vi "Timer.vi"(9 "Timer.Timer enable":bool, 10 "Timer.Tiempo deseado":dbl format="%#_13g", 11 "Class 2.lvclass":refnum<class "Class 2.lvclass">) -> (1 "Timer.Timer DN":bool, 2 "Numeric":dbl, 3 "Class 2.lvclass 2":refnum<class "Class 2.lvclass">)   [LabVIEW 2019, in "Class 2.lvclass"]
uses:
  Class 2.lvclass
  Class 2.lvclass/Class 2.ctl
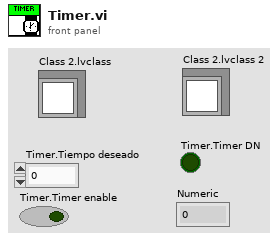
[diagram p1: front panel]
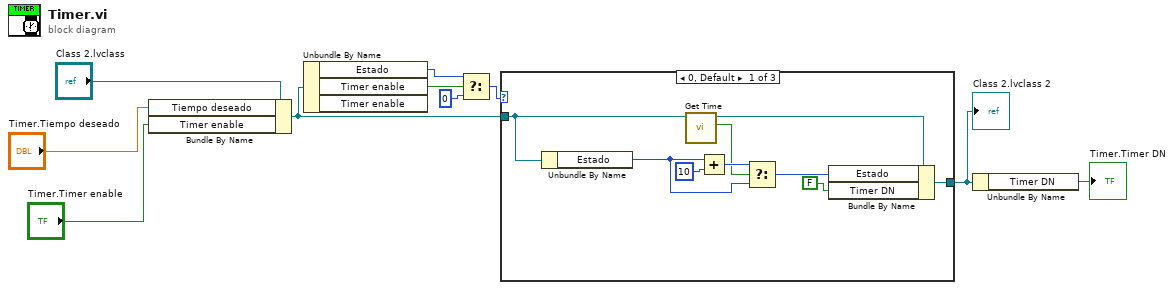
[diagram p0: block diagram]
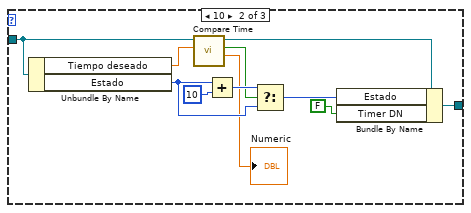
[diagram p2: hidden frame]
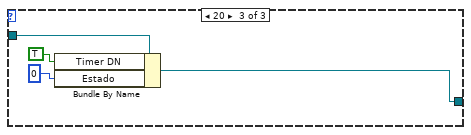
[diagram p3: hidden frame]
diagram:
  n1 = Bundle By Name(cluster="Class 2.lvclass", "Tiempo deseado"="Timer.Tiempo deseado", "Timer enable"="Timer.Timer enable") -> (w8:refnum<class "Class 2.lvclass">)
  n2 = Unbundle By Name(w8) -> ("Estado"=w4:u8, "Timer enable"=w3:bool)  [unwired: 1 out]
  n3 = Select(t=w4, s=w3, f=u8 0) -> (s? t:f=w1:u8)
  n4 = case shown="0, Default" w1 {
    tunnel: [w16 w24 w32] -> w9
    tunnel: w8 -> [w11 w20 w33]
    frame 0, Default {
      n5 = Unbundle By Name(w11) -> ("Estado"=w15:u8)
      n6 = call "Get Time.vi"("Class 2.lvclass"=w11) -> ("change"=w13:bool, "Class 2.lvclass 2"=w17:refnum<class "Class 2.lvclass">)  [unwired: 9 in]
      n7 = Add(x=w15, y=u8 10) -> (x+y=w18:u8)
      n8 = Select(t=w18, s=w13, f=w15) -> (s? t:f=w14:u8)
      n9 = Bundle By Name(cluster=w17, "Estado"=w14, "Timer DN"=FALSE ("Timer.Timer DN")) -> (w16:refnum<class "Class 2.lvclass">)
    }
    frame 10 {
      n10 = Unbundle By Name(w20) -> ("Tiempo deseado"=w26:dbl, "Estado"=w28:u8)
      n11 = call "Compare Time.vi"("TIEMPO DESEADO"=w26, "Class 2.lvclass"=w20) -> ("Numeric"=→"Numeric":dbl, "validacion"=w25:bool, "Class 2.lvclass 2"=w23:refnum<class "Class 2.lvclass">)  [unwired: 7 in]
      n12 = Add(x=w28, y=u8 10) -> (x+y=w29:u8)
      n13 = Select(t=w29, s=w25, f=w28) -> (s? t:f=w27:u8)
      n14 = Bundle By Name(cluster=w23, "Estado"=w27, "Timer DN"=FALSE ("Timer.Timer DN")) -> (w24:refnum<class "Class 2.lvclass">)
    }
    frame 20 {
      n15 = Bundle By Name(cluster=w33, "Timer DN"=TRUE ("Timer.Timer DN"), "Estado"=u8 0 ("Timer.Estado")) -> (w32:refnum<class "Class 2.lvclass">)
    }
  }
  "Class 2.lvclass 2" <- w9
  n16 = Unbundle By Name(w9) -> ("Timer DN"=→"Timer.Timer DN":bool)
